vi "pressure control advanced.vi"() -> ()   [LabVIEW 2013]
uses:
  <vilib>/Instr/_visa.llb/VISA Configure Serial Port (Instr).vi
panel:
  in  "% Open":dbl min=0.0 max=100.0 step=5.0
  in  "Butterfly Valve Control":enum32{"Valve Mode", "Pressure Mode"}(radio)
  in  "Torr":dbl min=0.0 max=760.0 step=5.0
  out "M106":string
  out "T40 or T51":string
  out "Valve position (%)":dbl
  out "Pressure (Torr)":dbl(graph)
  in  "stop":bool
  out "error out":errorcluster
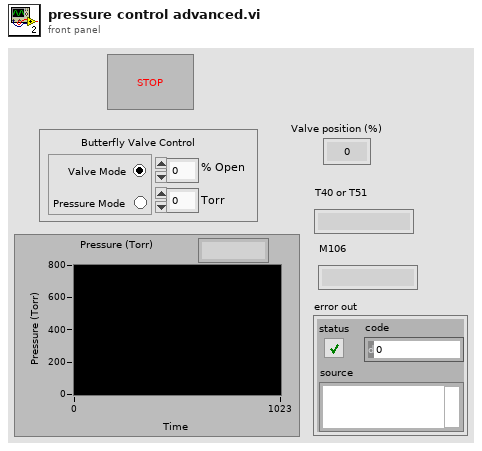
[diagram p1: front panel]
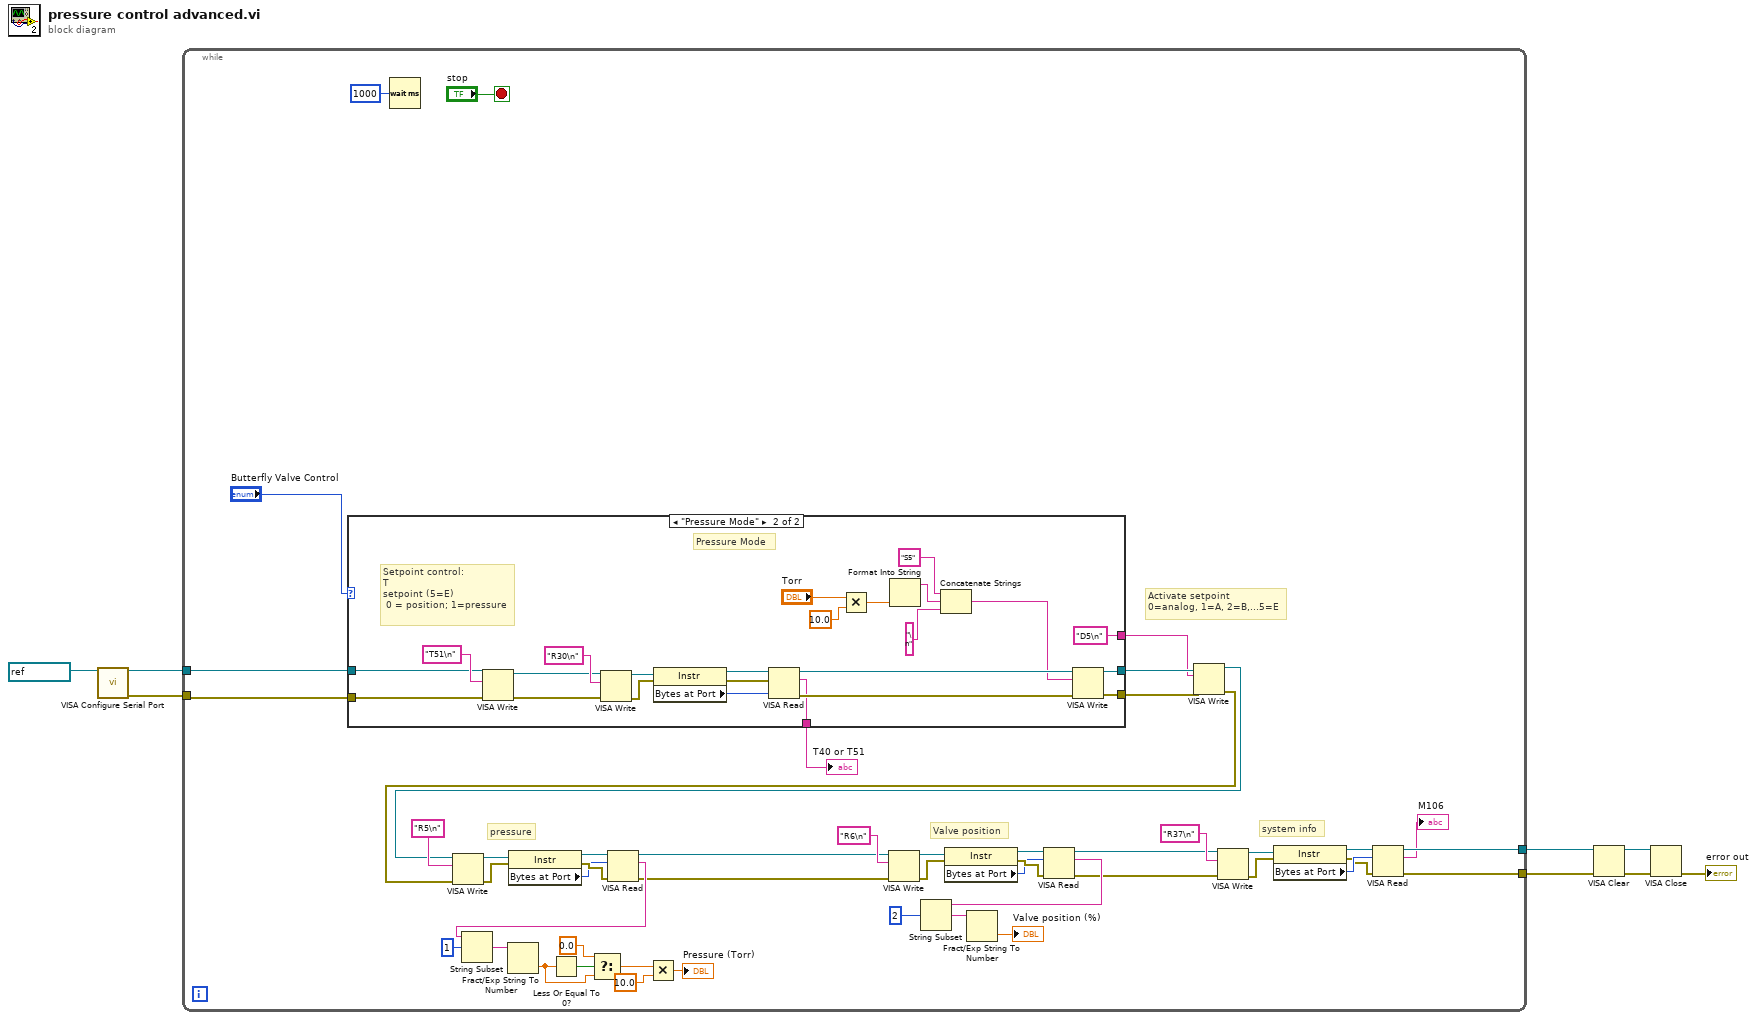
[diagram p0: block diagram]
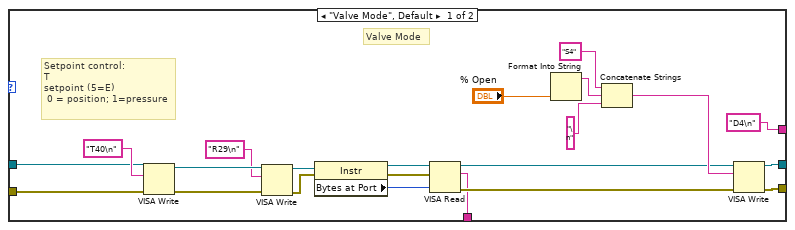
[diagram p2: hidden frame]
diagram:
  n1 = call-poly "VISA Configure Serial Port"("VISA resource name"=refnum<visa-resource-name> "COM5") -> ("VISA resource name out"=w7:refnum<visa-resource-name>, "error out"=w3:errorcluster)  [unwired: 13 in]
  n2 = while {
    tunnel: w7 -> [w18]
    tunnel: w3 -> [w17]
    tunnel: [w25] -> w2
    tunnel: [w24] -> w1
    stop <- "stop" stop-if-true
    # "system info"
    # "Activate setpoint \n0=analog, 1=A, 2=B,...5=E"
    # "pressure"
    # "Valve position"
    n3 = case shown="\"Pressure Mode\"" "Butterfly Valve Control" {
      tunnel: w18 -> [w63 w85]
      tunnel: w17 -> [w62 w86]
      tunnel: [w61 w88] -> w16
      tunnel: [w60 w87] -> w15
      tunnel: [w59 w84] -> w14
      tunnel: ["D4\n" ("write buffer") "D5\n" ("write buffer")] -> w12
      frame "Valve Mode", Default {
        # "Valve Mode"
        # "Setpoint control:\nT\nsetpoint (5=E)\n 0 = position; 1=pressure"
        n4 = VISA Write(VISA resource name=w63, write buffer="T40\n", error in (no error)=w62) -> (VISA resource name out=w74:refnum<visa-resource-name>, error out=w72:errorcluster)  [unwired: 1 out]
        n5 = VISA Write(VISA resource name=w74, write buffer="R29\n", error in (no error)=w72) -> (VISA resource name out=w67:refnum<visa-resource-name>, error out=w68:errorcluster)  [unwired: 1 out]
        n6 = property class="Instr"(reference=w67, error in=w68) -> (reference out=w65:refnum<visa-resource-name>, error out=w66:errorcluster, "Bytes at Port"=w73:u32)
        n7 = VISA Read(VISA resource name=w65, byte count=w73, error in (no error)=w66) -> (VISA resource name out=w71:refnum<visa-resource-name>, read buffer=w59:string, error out=w70:errorcluster)  [unwired: 1 out]
        n8 = Format Into String("% Open") -> (resulting string=w79:string)  [unwired: 3 in, 1 out]
        n9 = Concatenate Strings("S4" ("string"), w79, "\n" ("string")) -> (w76:string)
        n10 = VISA Write(VISA resource name=w71, write buffer=w76, error in (no error)=w70) -> (VISA resource name out=w61:refnum<visa-resource-name>, error out=w60:errorcluster)  [unwired: 1 out]
      }
      frame "Pressure Mode" {
        # "Pressure Mode"
        # "Setpoint control:\nT\nsetpoint (5=E)\n 0 = position; 1=pressure"
        n11 = VISA Write(VISA resource name=w85, write buffer="T51\n", error in (no error)=w86) -> (VISA resource name out=w93:refnum<visa-resource-name>, error out=w95:errorcluster)  [unwired: 1 out]
        n12 = VISA Write(VISA resource name=w93, write buffer="R30\n", error in (no error)=w95) -> (VISA resource name out=w100:refnum<visa-resource-name>, error out=w99:errorcluster)  [unwired: 1 out]
        n13 = property class="Instr"(reference=w100, error in=w99) -> (reference out=w102:refnum<visa-resource-name>, error out=w101:errorcluster, "Bytes at Port"=w94:u32)
        n14 = VISA Read(VISA resource name=w102, byte count=w94, error in (no error)=w101) -> (VISA resource name out=w96:refnum<visa-resource-name>, read buffer=w84:string, error out=w97:errorcluster)  [unwired: 1 out]
        n15 = Multiply(x="Torr", y=10.0) -> (x*y=w80:dbl)
        n16 = Format Into String(w80) -> (resulting string=w89:string)  [unwired: 3 in, 1 out]
        n17 = Concatenate Strings("S5" ("string"), w89, "\n" ("string")) -> (w91:string)
        n18 = VISA Write(VISA resource name=w96, write buffer=w91, error in (no error)=w97) -> (VISA resource name out=w88:refnum<visa-resource-name>, error out=w87:errorcluster)  [unwired: 1 out]
      }
    }
    "T40 or T51" <- w14
    n19 = Wait (ms)(milliseconds to wait=u32 1000) -> ()  [unwired: 1 out]
    n20 = VISA Write(VISA resource name=w16, write buffer=w12, error in (no error)=w15) -> (VISA resource name out=w20:refnum<visa-resource-name>, error out=w22:errorcluster)  [unwired: 1 out]
    n21 = VISA Write(VISA resource name=w20, write buffer="R5\n", error in (no error)=w22) -> (VISA resource name out=w43:refnum<visa-resource-name>, error out=w42:errorcluster)  [unwired: 1 out]
    n22 = property class="Instr"(reference=w43, error in=w42) -> (reference out=w46:refnum<visa-resource-name>, error out=w45:errorcluster, "Bytes at Port"=w44:u32)
    n23 = VISA Read(VISA resource name=w46, byte count=w44, error in (no error)=w45) -> (VISA resource name out=w35:refnum<visa-resource-name>, read buffer=w39:string, error out=w34:errorcluster)  [unwired: 1 out]
    n24 = String Subset(string=w39, offset (0)=1) -> (substring=w41:string)  [unwired: 1 in]
    n25 = Fract/Exp String To Number(string=w41) -> (number=w36:dbl)  [unwired: 3 in, 1 out]
    n26 = Less Or Equal To 0?(x=w36) -> (x <= 0?=w38:bool)
    n27 = Select(t=0.0, s=w38, f=w36) -> (s? t:f=w10:dbl)
    n28 = Multiply(x=w10, y=10.0) -> (x*y=→"Pressure (Torr)":dbl)
    n29 = VISA Write(VISA resource name=w35, write buffer="R6\n", error in (no error)=w34) -> (VISA resource name out=w52:refnum<visa-resource-name>, error out=w51:errorcluster)  [unwired: 1 out]
    n30 = property class="Instr"(reference=w52, error in=w51) -> (reference out=w55:refnum<visa-resource-name>, error out=w54:errorcluster, "Bytes at Port"=w53:u32)
    n31 = VISA Read(VISA resource name=w55, byte count=w53, error in (no error)=w54) -> (VISA resource name out=w27:refnum<visa-resource-name>, read buffer=w50:string, error out=w26:errorcluster)  [unwired: 1 out]
    n32 = String Subset(string=w50, offset (0)=2) -> (substring=w48:string)  [unwired: 1 in]
    n33 = Fract/Exp String To Number(string=w48) -> (number=→"Valve position (%)":dbl)  [unwired: 3 in, 1 out]
    n34 = VISA Write(VISA resource name=w27, write buffer="R37\n", error in (no error)=w26) -> (VISA resource name out=w32:refnum<visa-resource-name>, error out=w33:errorcluster)  [unwired: 1 out]
    n35 = property class="Instr"(reference=w32, error in=w33) -> (reference out=w29:refnum<visa-resource-name>, error out=w30:errorcluster, "Bytes at Port"=w31:u32)
    n36 = VISA Read(VISA resource name=w29, byte count=w31, error in (no error)=w30) -> (VISA resource name out=w24:refnum<visa-resource-name>, read buffer=→"M106":string, error out=w25:errorcluster)  [unwired: 1 out]
  }
  n37 = VISA Clear(VISA resource name=w1, error in (no error)=w2) -> (VISA resource name out=w6:refnum<visa-resource-name>, error out=w5:errorcluster)
  n38 = VISA Close(VISA resource name=w6, error in (no error)=w5) -> (error out=→"error out":errorcluster)
